vi "PressureGroups2Calibrate.vi"(9 "Valves":u16[](array[ring]) items=["A1", "A2", "A3", "A4", "B1", "B2", "B3", "B4", "B5", "B6", "B7", "B8", "A5"], 10 "Pressure Group":enum16{"1", "2", "3", "4"}[](array[ring])=[enum."3", enum."3", enum."3", enum."3", enum."4", enum."4", enum."4", enum."4", enum."1", enum."1", enum."1", enum."1", enum."1"], 11 "Mix Sequence Array":bool[][](array[boolean])) -> (2 "Valves 2 Calibrate":u16[](array[ring]) items=["A1", "A2", "A3", "A4", "B1", "B2", "B3", "B4", "B5", "B6", "B7", "B8", "A5"], 3 "Pressure Groups to Calibrate":u16[](array[numeric])=[2, 2, 2, 2, 3, 3, 3, 3, 0, 0, 0, 0, 0])   [LabVIEW 2016]
uses:
  <vilib>/imath/engines/lvmath2/RunTimeEngine/BuiltInFunctions/any/NIMS_any(GM).vi
  <vilib>/imath/engines/lvmath2/RunTimeEngine/VariableToken/Support/NIMS_Matrix Boolean Index to I32 Index.vi
  <vilib>/imath/engines/lvmath2/RunTimeEngine/IndexRead/NIMS V(V).vi
  <instcachedir>/0/NIMS V(V)_298D9CB7BFEB42B8BC8D9C3C28AE8C70.lvgen/NIMS V(V)_298D9CB7BFEB42B8BC8D9C3C28AE8C70_001.vi
  <vilib>/imath/engines/lvmath2/RunTimeEngine/BuiltInFunctions/sets_unique/NIMS_sets_unique(GV).vi
  <instcachedir>/0/NIMS_sets_unique(GV)_BC60CBD939E647F382369330BF9EA64D.lvgen/NIMS_sets_unique(GV)_BC60CBD939E647F382369330BF9EA64D_006.vi
  <vilib>/imathl/engines/lvmath/Functions/Error Handling/Create Error.vi
  <vilib>/imath/engines/lvmath2/RunTimeEngine/BuiltInFunctions/length/NIMS_length(GV).vi
  <instcachedir>/0/NIMS_length(GV)_08A3D13377FD4E4B96F5795FBF3698FA.lvgen/NIMS_length(GV)_08A3D13377FD4E4B96F5795FBF3698FA_003.vi
  <vilib>/imath/engines/lvmath2/RunTimeEngine/RangeToken/NIMS_Range_R2 - Integer.vi
  <instcachedir>/0/NIMS_Range_R2 - Integer_416A044C4F024DBE8E97DA138CB3186F.lvgen/NIMS_Range_R2 - Integer_416A044C4F024DBE8E97DA138CB3186F_000.vi
  <vilib>/imath/engines/lvmath2/RunTimeEngine/CommandStatement/MC_CommandStatement_break.vi
  <vilib>/imath/engines/lvmath2/RunTimeEngine/IndexRead/NIMS V(S).vi
  <instcachedir>/0/NIMS V(S)_0488751826AF41519A22953C041130DC.lvgen/NIMS V(S)_0488751826AF41519A22953C041130DC_003.vi
  <vilib>/imath/engines/lvmath2/RunTimeEngine/BuiltInFunctions/findnz/NIMS_[1o]_findnz(GRowV).vi
  <instcachedir>/0/NIMS_[1o]_findnz(GRowV)_656056C849EF4762B1F0843BDDDEF2FF.lvgen/NIMS_[1o]_findnz(GRowV)_656056C849EF4762B1F0843BDDDEF2FF_000.vi
  <vilib>/imath/engines/lvmath2/RunTimeEngine/VariableToken/NIMS_VariableToken_CondDefinedDefinedByReplace.vi
  <instcachedir>/0/NIMS_VariableToken_CondDefinedDefinedByReplace_D162CFFC24174562A9FEA619A91E1A56.lvgen/NIMS_VariableToken_CondDefinedDefinedByReplace_D162CFFC24174562A9FEA619A91E1A56_003.vi
  <vilib>/imath/engines/lvmath2/RunTimeEngine/IndexReplace/NIMS V(S)=V.vi
  <instcachedir>/0/NIMS V(S)=V_16451AC3E73743A5BCE8279D025B19B1.lvgen/NIMS V(S)=V_16451AC3E73743A5BCE8279D025B19B1_001.vi
  <vilib>/imath/engines/lvmath2/RunTimeEngine/ErrorHandling/NIMS_Create Error From Enums.vi
  <vilib>/imath/engines/lvmath2/RunTimeEngine/VariableToken/NIMS_VariableToken_CondDefined.vi
  <instcachedir>/0/NIMS_VariableToken_CondDefined_620A15720FCC4DA7863546285C12295E.lvgen/NIMS_VariableToken_CondDefined_620A15720FCC4DA7863546285C12295E_004.vi
  <vilib>/imath/engines/lvmath/Functions/Error Handling/MergeErrorsWrapper.vi
  <vilib>/imath/engines/lvmath2/RunTimeEngine/NodeEndStatement/NIMS_NodeEndStatement_Output.vi
  <instcachedir>/0/NIMS_NodeEndStatement_Output_53EC0D466D134D7ABD903AC30B43404B.lvgen/NIMS_NodeEndStatement_Output_53EC0D466D134D7ABD903AC30B43404B_011.vi
  <vilib>/imath/engines/lvmath2/RunTimeEngine/ErrorHandling/NIMS_Finalize Error.vi
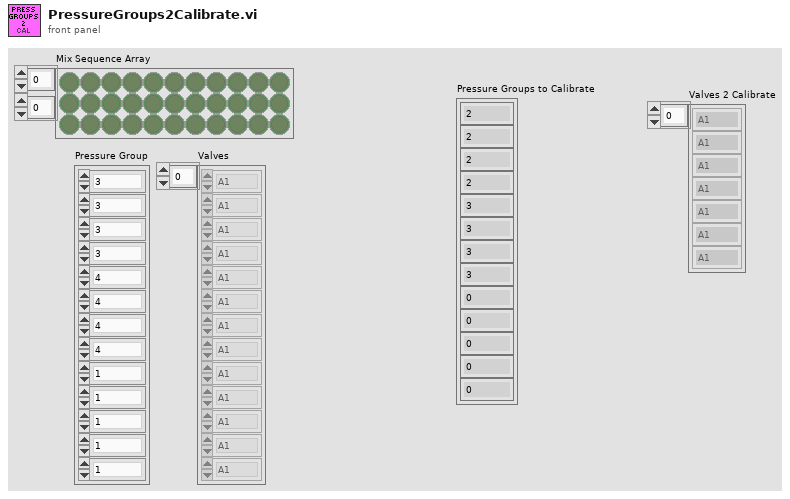
[diagram p1: front panel]
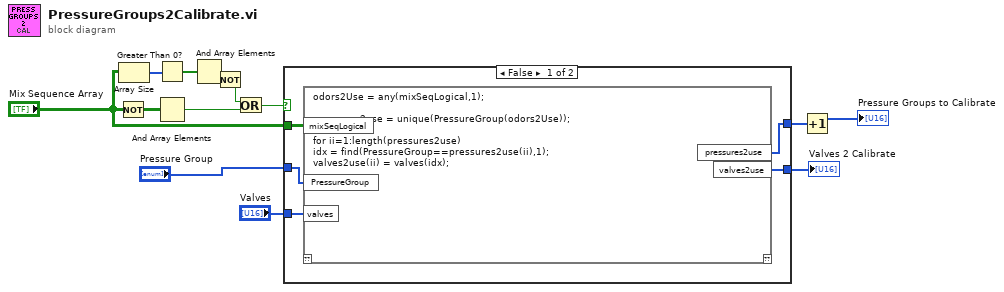
[diagram p0: block diagram]
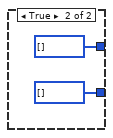
[diagram p2: hidden frame]
diagram:
  n1 = Not(x="Mix Sequence Array") -> (.not. x?=w6:bool[][])
  n2 = Array Size(array="Mix Sequence Array") -> (size(s)=w9:i32[])
  n3 = Greater Than 0?(x=w9) -> (x > 0?=w8:bool[])
  n4 = And Array Elements(Boolean array=w6) -> (logical AND=w3:bool)
  n5 = And Array Elements(Boolean array=w8) -> (logical AND=w5:bool)
  n6 = Not(x=w5) -> (.not. x?=w2:bool)
  n7 = Or(x=w2, y=w3) -> (x .or. y?=w4:bool)
  n8 = case shown="False" w4 {
    tunnel: "Pressure Group" -> [w18 _]
    tunnel: [w17 u16[] [] ("pressures2use")] -> w12
    tunnel: [w16 u16[] [] ("valves2use")] -> w11
    tunnel: "Valves" -> [w15 _]
    tunnel: "Mix Sequence Array" -> [w14 _]
    frame False {
      n9 = mathscript code="odors2Use = any(mixSeqLogical,1);\n\npressures2use = unique(PressureGroup(odors2Use));\n\nfor ii=1:length(pressures2use)\nidx = find(PressureGroup==pressures2use(ii),1);\nvalves2use(ii) = valves(idx);\n\nend"("mixSeqLogical"=w14, "PressureGroup"=w18, "valves"=w15) -> ("valves2use"=w16:u16[], "pressures2use"=w17:u16[])  [unwired: 1 in, 1 out]
    }
    frame True {
    }
  }
  "Valves 2 Calibrate" <- w11
  n10 = Increment(x=w12) -> (x+1=→"Pressure Groups to Calibrate":u16[])
